vi "emi_SMLoop Start.vi"(5 "Loop ID":i32, 9 "error in (no error)":errorcluster, 12 "Force Stop(F)":bool) -> (6 "Loop command":T1, 10 "error out":errorcluster, 14 "Loop ID out":i32)   [LabVIEW 2011]
uses:
  Private/_emi_ SMLoop sates.ctl
  Loop control/Private/_emi_Loop control int action.ctl
  Private/_emi_ SMLoop restart type.ctl
  S&E reporting/emi_Send S&E Error message.vi
  Basic/0 - General/Error/emi_ Is Error state.vi
  emi_Read System ID.vi
  Private/_emi_GFV System ID.vi
  S&E reporting/Private/_emi_S&E Q Generator.vi
  Loop control/Private/_emi_GFV stop a loop so it can reset.vi
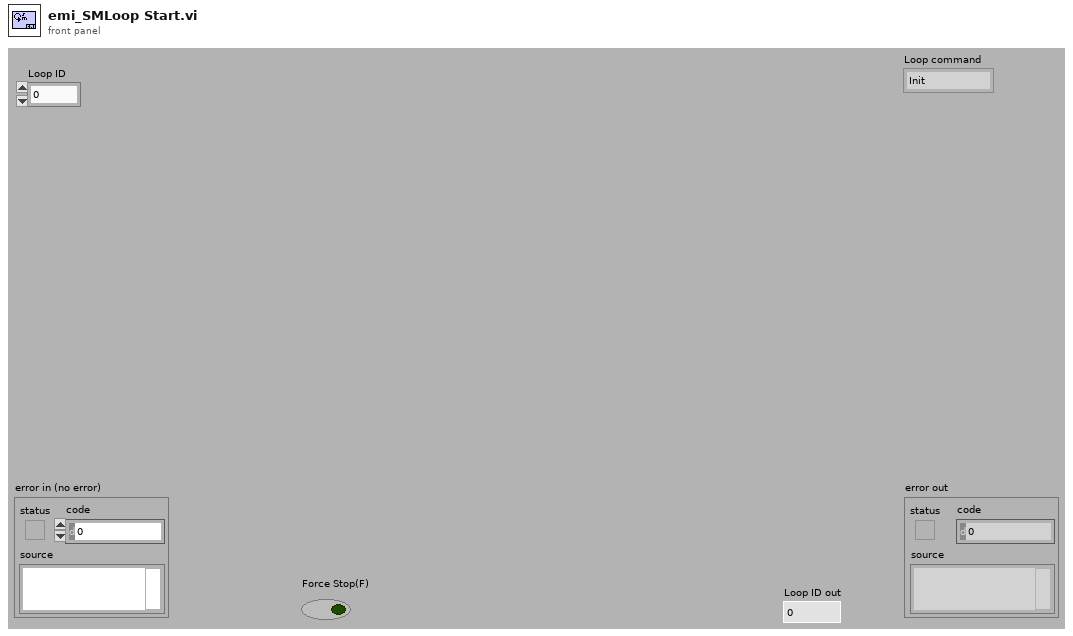
[diagram p1: front panel]
types:
  T1 = typedef "_emi_ SMLoop sates.ctl" = enum16{"Init", "Standby", "Start", "Normal Operation", "Stop", "Error Handling", "End", "Post"}
  T2 = typedef "_emi_ SMLoop restart type.ctl" = enum16{"Normal", "Stop", "Stopped"}
  T3 = typedef "_emi_Loop control int action.ctl" = enum16{"Init index", "Get index", "Set index", "Get Size"}
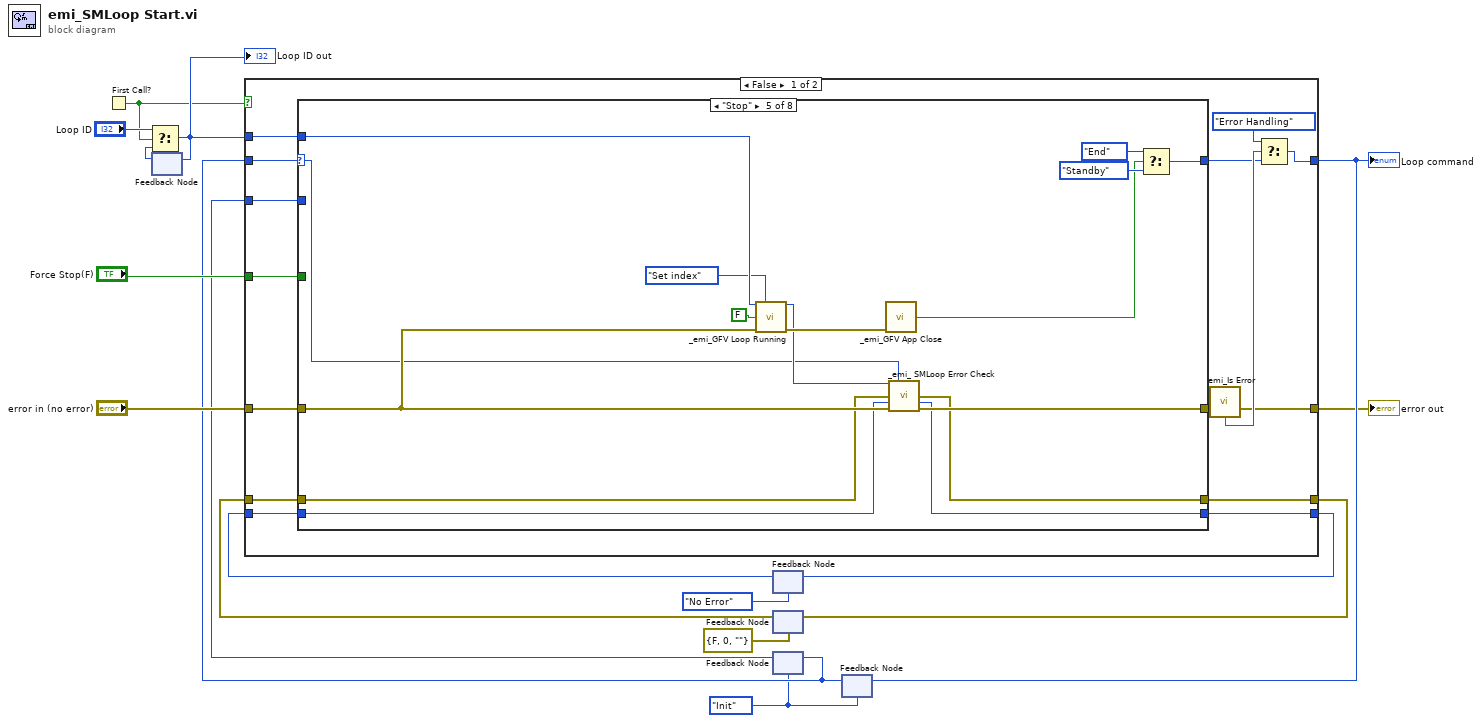
[diagram p0: block diagram]
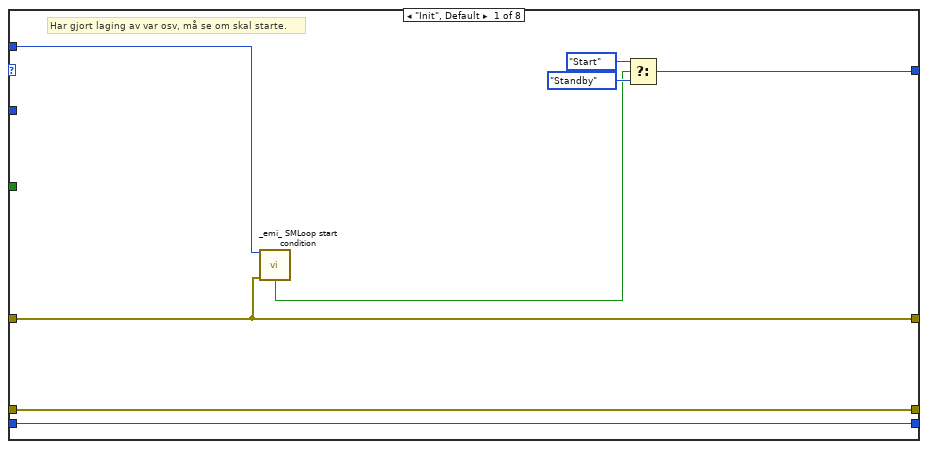
[diagram p2: hidden frame]
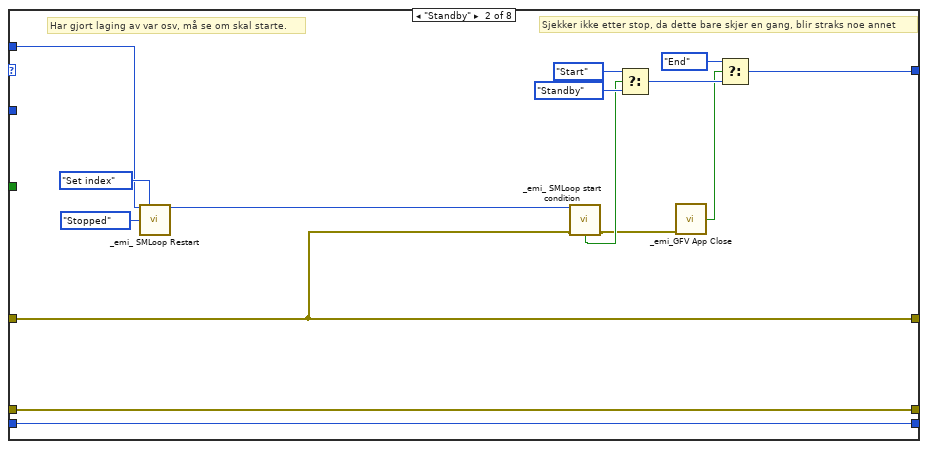
[diagram p3: hidden frame]
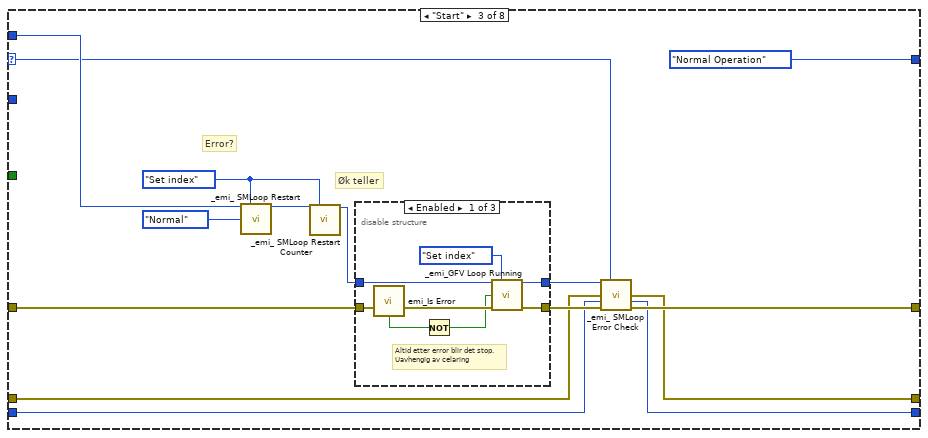
[diagram p4: hidden frame]
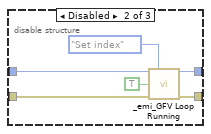
[diagram p5: hidden frame]
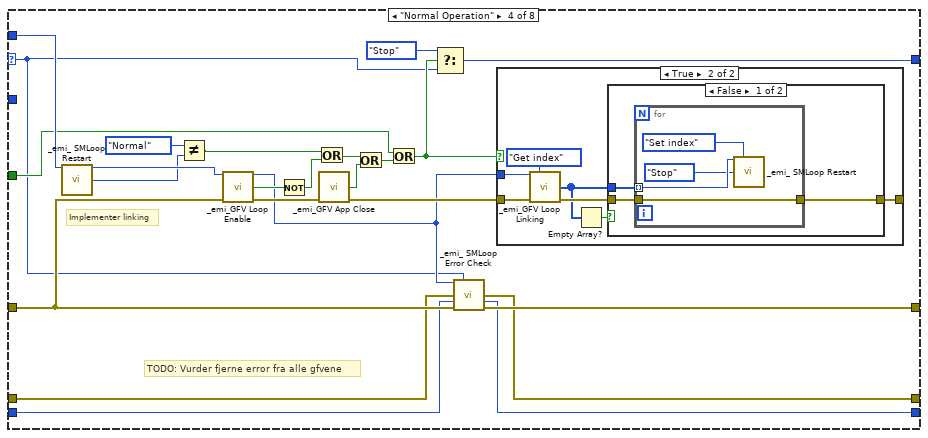
[diagram p7: hidden frame]
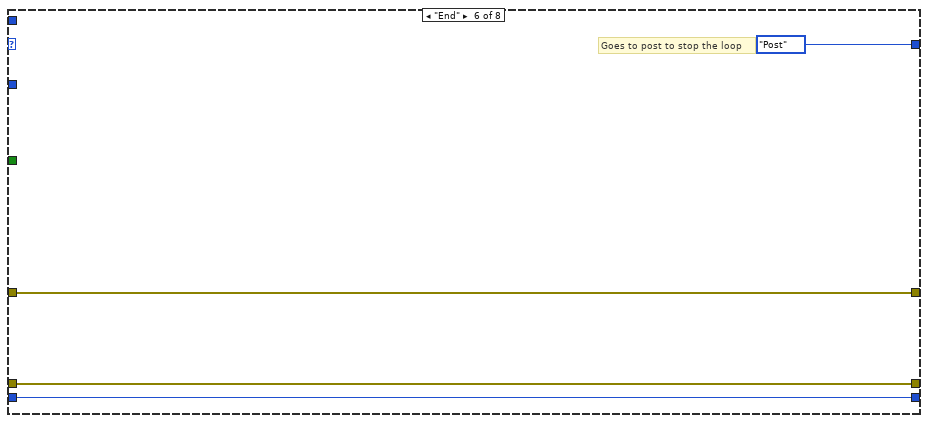
[diagram p10: hidden frame]
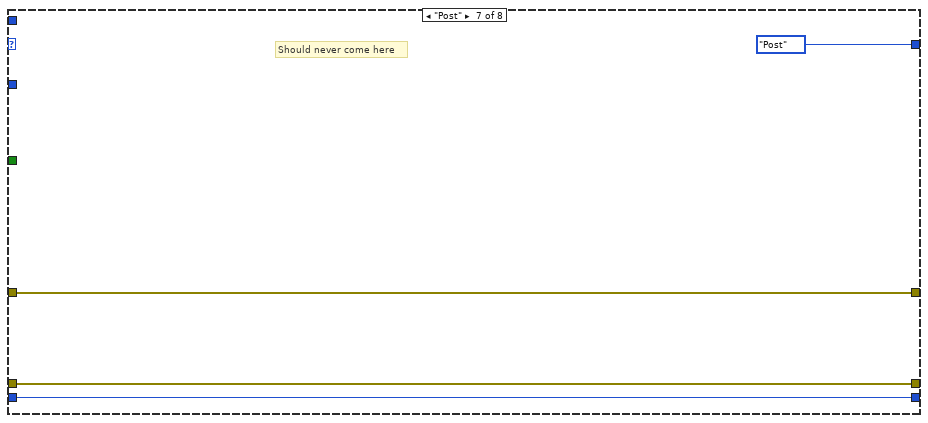
[diagram p11: hidden frame]
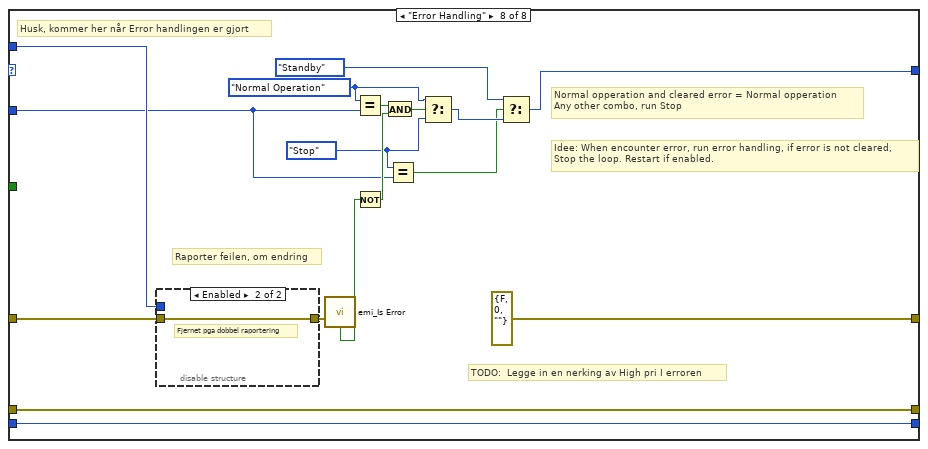
[diagram p12: hidden frame]
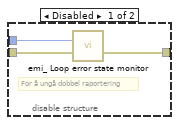
[diagram p13: hidden frame]
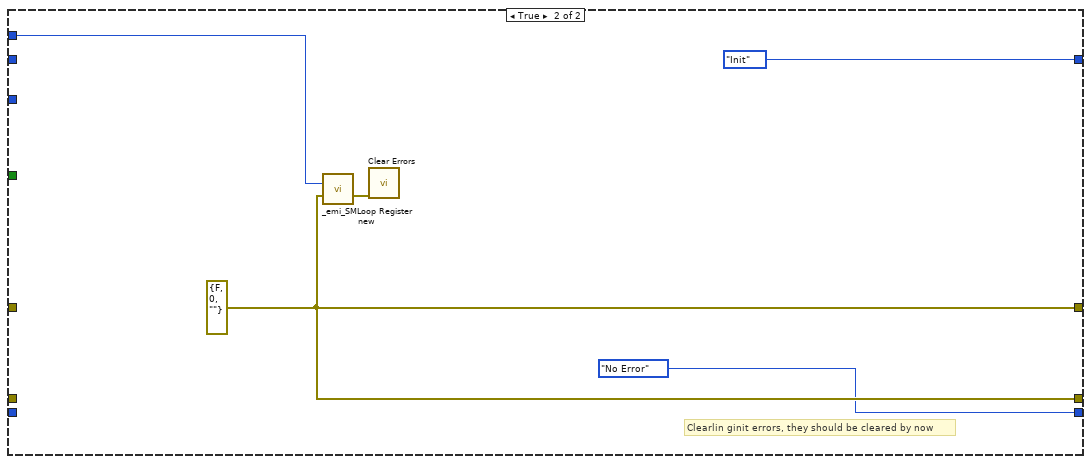
[diagram p14: hidden frame]
diagram:
  w7 = _emi__SMLoop_sates."Init" ("Loop command")
  n1 = First Call?() -> (First Call?: T/F=w13:bool)
  n2 = feedback #1() -> (w17:i32)  [unwired: 1 in]
  n3 = Select(t="Loop ID", s=w13, f=w17) -> (s? t:f=w14:i32)
  "Loop ID out" <- w14
  n4 = feedback-in #1(w14) -> ()
  n5 = feedback #2(enum16{"No Error", "Start", "Normal", "Stop"}."No Error" ("Source Out")) -> (w3:enum16{"No Error", "Start", "Normal", "Stop"})
  n6 = feedback #3(errorcluster {"status"=FALSE, "code"=0, "source"=""} ("Loop Error state out")) -> (w4:errorcluster)
  n7 = feedback #4(w7) -> (w8:T1)
  n8 = feedback #5(w7) -> (w9:T1)
  n9 = case shown="False" w13 {
    tunnel: [w26 _emi__SMLoop_sates."Init" ("Loop command")] -> w16
    tunnel: w9 -> [w22 _]
    tunnel: w14 -> [w31 w175]
    tunnel: [w23 w173] -> w12
    tunnel: "error in (no error)" -> [w32 _]
    tunnel: "Force Stop(F)" -> [w30 _]
    tunnel: w8 -> [w29 _]
    tunnel: [w21 w173] -> w6
    tunnel: [w20 enum16{"No Error", "Start", "Normal", "Stop"}."No Error" ("Source Out")] -> w5
    tunnel: w4 -> [w19 _]
    tunnel: w3 -> [w18 _]
    frame False {
      n10 = case shown="\"Stop\"" w22 {
        selector: w22 -> [_ _ w64 w87 w127 _ _ _]
        tunnel: [w35 w46 w65 w93 w133 w146 w150 errorcluster {"status"=FALSE, "code"=0, "source"=""} ("error out")] -> w24
        tunnel: w32 -> [w35 w46 w68 w94 w134 w146 w150 w167]
        tunnel: [w39 w53 _emi__SMLoop_sates."Normal Operation" ("t") w102 w142 _emi__SMLoop_sates."Post" ("t") _emi__SMLoop_sates."Post" ("t") w155] -> w25
        tunnel: w31 -> [w37 w47 w67 w101 w137 _ _ w164]
        tunnel: w30 -> [_ _ _ w95 _ _ _ _]
        tunnel: w29 -> [_ _ _ _ _ _ _ w154]
        tunnel: [w34 w42 w62 w89 w129 w144 w148 w152] -> w21
        tunnel: [w33 w41 w61 w91 w130 w143 w147 w151] -> w20
        tunnel: w19 -> [w34 w42 w59 w90 w131 w144 w148 w152]
        tunnel: w18 -> [w33 w41 w60 w92 w132 w143 w147 w151]
        frame "Init", Default {
          # "Har gjort laging av var osv, må se om skal starte."
          n11 = call "_emi_ SMLoop start condition.vi"("Loop ID in"=w37, "error in (no error)"=w35) -> ("Klar til start"=w36:bool)  [unwired: 11 in, 2 out]
          n12 = Select(t=_emi__SMLoop_sates."Start", s=w36, f=_emi__SMLoop_sates."Standby") -> (s? t:f=w39:T1)
        }
        frame "Standby" {
          # "Sjekker ikke etter stop, da dette bare skjer en gang, blir straks noe annet"
          # "Har gjort laging av var osv, må se om skal starte."
          n13 = call "_emi_ SMLoop Restart.vi"("Loop Index/Numb"=w47, "Action(Get Index)"=_emi_Loop_control_int_action."Set index", "Value"=_emi__SMLoop_restart_type."Stopped") -> ("Index out"=w45:u16)  [unwired: 10 in, 2 out]
          n14 = call "_emi_ SMLoop start condition.vi"("Loop ID in"=w45, "error in (no error)"=w46) -> ("Klar til start"=w44:bool, "error out"=w43:errorcluster)  [unwired: 11 in, 1 out]
          n15 = Select(t=_emi__SMLoop_sates."Start", s=w44, f=_emi__SMLoop_sates."Standby") -> (s? t:f=w52:T1)
          n16 = call "_emi_GFV App Close.vi"("error in (no error)"=w43) -> ("App Close out"=w50:bool)  [unwired: 13 in, 1 out]
          n17 = Select(t=_emi__SMLoop_sates."End", s=w50, f=w52) -> (s? t:f=w53:T1)
        }
        frame "Start" {
          w56 = _emi_Loop_control_int_action."Set index" ("Action(Get Index)")
          # "Øk teller"
          # "Error?"
          n18 = call "_emi_ SMLoop Restart.vi"("Loop Index/Numb"=w67, "Action(Get Index)"=w56, "Value"=_emi__SMLoop_restart_type."Normal") -> ("Index out"=w58:u16)  [unwired: 10 in, 2 out]
          n19 = call "_emi_ SMLoop Restart Counter.vi"("Loop Index/Numb"=w58, "Action(Get Index)"=w56) -> ("Index out"=w57:u16)  [unwired: 11 in, 2 out]
          n20 = disable-structure shown="Enabled" {
            disable-tunnel: w68 -> [w74 w84 w86]
            disable-tunnel: [w78 w81 w86] -> w66
            disable-tunnel: [w77 w80 w85] -> w63
            disable-tunnel: w57 -> [w76 w79 w85]
            frame Enabled {
              # "Altid etter error blir det stop.\nUavhengig av celaring"
              n21 = call "emi_Is Error.vi"("error in (no error)"=w74) -> ("error out"=w72:errorcluster, "Is Error"=w73:bool)  [unwired: 13 in]
              n22 = Not(x=w73) -> (.not. x?=w71:bool)
              n23 = call "_emi_GFV Loop Running.vi"("Loop Index/Numb"=w76, "Action(Get Index)"=_emi_Loop_control_int_action."Set index", "Loop Running In(F)"=w71, "error in (no error)"=w72) -> ("Index out"=w77:u16, "error out"=w78:errorcluster)  [unwired: 8 in, 2 out]
            }
            frame Disabled {
              n24 = call "_emi_GFV Loop Running.vi"("Loop Index/Numb"=w79, "Action(Get Index)"=_emi_Loop_control_int_action."Set index", "Loop Running In(F)"=TRUE, "error in (no error)"=w84) -> ("Index out"=w80:u16, "error out"=w81:errorcluster)  [unwired: 8 in, 2 out]
            }
            frame Disabled {
              # "Viste Connected når restartet på feil"
            }
          }
          n25 = call "_emi_ SMLoop Error Check.vi"("Loop Index"=w63, "Command ID"=w64, "Loop  Current Error State"=w59, "Current Loop Error/Warning Source"=w60, "Error in"=w66) -> ("Loop Error state out"=w62:errorcluster, "Source Out"=w61:enum16{"No Error", "Start", "Normal", "Stop"}, "error out"=w65:errorcluster)  [unwired: 7 in, 1 out]
        }
        frame "Normal Operation" {
          # "TODO: Vurder fjerne error fra alle gfvene"
          # "Implementer linking"
          n26 = call "_emi_ SMLoop Restart.vi"("Loop Index/Numb"=w101) -> ("Index out"=w100:u16, "Value out"=w98:T2)  [unwired: 12 in, 1 out]
          n27 = Not Equal?(x=_emi__SMLoop_restart_type."Normal", y=w98) -> (x != y?=w99:bool)
          n28 = call "_emi_GFV Loop Enable.vi"("Loop Index/Numb"=w100, "error in (no error)"=w94) -> ("Index out"=w88:u16, "Loop Enable Out"=w107:bool, "error out"=w109:errorcluster)  [unwired: 10 in, 1 out]
          n29 = Not(x=w107) -> (.not. x?=w105:bool)
          n30 = Or(x=w99, y=w105) -> (x .or. y?=w106:bool)
          n31 = call "_emi_GFV App Close.vi"("error in (no error)"=w109) -> ("App Close out"=w110:bool, "error out"=w96:errorcluster)  [unwired: 13 in]
          n32 = Or(x=w106, y=w110) -> (x .or. y?=w108:bool)
          n33 = Or(x=w95, y=w108) -> (x .or. y?=w103:bool)
          n34 = Select(t=_emi__SMLoop_sates."Stop", s=w103, f=w87) -> (s? t:f=w102:T1)
          n35 = call "_emi_ SMLoop Error Check.vi"("Loop Index"=w88, "Command ID"=w87, "Loop  Current Error State"=w90, "Current Loop Error/Warning Source"=w92, "Error in"=w94) -> ("Loop Error state out"=w89:errorcluster, "Source Out"=w91:enum16{"No Error", "Start", "Normal", "Stop"}, "error out"=w93:errorcluster)  [unwired: 7 in, 1 out]
          n36 = case shown="True" w103 {
            tunnel: [w111 w114] -> _
            tunnel: w96 -> [w111 w113]
            tunnel: w88 -> [_ w112]
            frame False {
            }
            frame True {
              n37 = call "_emi_GFV Loop Linking.vi"("Loop Index/Numb"=w112, "Action(Get Index)"=_emi_Loop_control_int_action."Get index", "error in (no error)"=w113) -> ("Linked indexes out"=w115:u16[], "error out"=w116:errorcluster)  [unwired: 9 in, 2 out]
              n38 = Empty Array?(array=w115) -> (empty?=w117:bool)
              n39 = case shown="False" w117 {
                tunnel: w116 -> [w121 w126]
                tunnel: [w120 w126] -> w114
                tunnel: w115 -> [w119 _]
                frame False {
                  n40 = for {
                    tunnel: w121 -> [w124]
                    tunnel: [w124] -> w120
                    tunnel: w119 -> [w123] mode=indexing
                    n41 = call "_emi_ SMLoop Restart.vi"("Loop Index/Numb"=w123, "Action(Get Index)"=_emi_Loop_control_int_action."Set index", "Value"=_emi__SMLoop_restart_type."Stop") -> ()  [unwired: 10 in, 3 out]
                  }
                }
                frame True {
                  # "Empty"
                }
              }
            }
          }
        }
        frame "Stop" {
          n42 = call "_emi_GFV Loop Running.vi"("Loop Index/Numb"=w137, "Action(Get Index)"=_emi_Loop_control_int_action."Set index", "Loop Running In(F)"=FALSE, "error in (no error)"=w134) -> ("Index out"=w128:u16, "error out"=w135:errorcluster)  [unwired: 8 in, 2 out]
          n43 = call "_emi_GFV App Close.vi"("error in (no error)"=w135) -> ("App Close out"=w139:bool)  [unwired: 13 in, 1 out]
          n44 = call "_emi_ SMLoop Error Check.vi"("Loop Index"=w128, "Command ID"=w127, "Loop  Current Error State"=w131, "Current Loop Error/Warning Source"=w132, "Error in"=w134) -> ("Loop Error state out"=w129:errorcluster, "Source Out"=w130:enum16{"No Error", "Start", "Normal", "Stop"}, "error out"=w133:errorcluster)  [unwired: 7 in, 1 out]
          n45 = Select(t=_emi__SMLoop_sates."End", s=w139, f=_emi__SMLoop_sates."Standby") -> (s? t:f=w142:T1)
        }
        frame "End" {
          # "Goes to post to stop the loop"
        }
        frame "Post" {
          # "Should never come here"
        }
        frame "Error Handling" {
          w159 = _emi__SMLoop_sates."Stop" ("f")
          w158 = _emi__SMLoop_sates."Normal Operation" ("x")
          # "Husk, kommer her når Error handlingen er gjort"
          # "Raporter feilen, om endring"
          # "TODO:  Legge in en nerking av High pri I erroren"
          # "Idee: When encounter error, run error handling, if error is not cleared,\nStop the loop. Restart if enabled."
          # "Normal opperation and cleared error = Normal opperation\nAny other combo, run Stop"
          n46 = disable-structure shown="Enabled" {
            disable-tunnel: w167 -> [w170 w171]
            disable-tunnel: [w169 w171] -> w165
            disable-tunnel: w164 -> [w168 _]
            frame Disabled {
              # "For å ungå dobbel raportering"
              n47 = call "emi_ Loop error state monitor.vi"("Loop ID in"=w168, "error in (no error)"=w170) -> ("error out"=w169:errorcluster)  [unwired: 12 in, 1 out]
            }
            frame Enabled {
              # "Fjernet pga dobbel raportering"
            }
          }
          n48 = call "emi_Is Error.vi"("error in (no error)"=w165) -> ("Is Error"=w153:bool)  [unwired: 13 in, 1 out]
          n49 = Equal?(x=w158, y=w154) -> (x = y?=w157:bool)
          n50 = Not(x=w153) -> (.not. x?=w160:bool)
          n51 = And(x=w157, y=w160) -> (x .and. y?=w156:bool)
          n52 = Equal?(x=w159, y=w154) -> (x = y?=w161:bool)
          n53 = Select(t=w158, s=w156, f=w159) -> (s? t:f=w162:T1)
          n54 = Select(t=_emi__SMLoop_sates."Standby", s=w161, f=w162) -> (s? t:f=w155:T1)
        }
      }
      n55 = call "emi_Is Error.vi"("error in (no error)"=w24) -> ("error out"=w23:errorcluster, "Is Error"=w27:bool)  [unwired: 13 in]
      n56 = Select(t=_emi__SMLoop_sates."Error Handling", s=w27, f=w25) -> (s? t:f=w26:T1)
    }
    frame True {
      w173 = errorcluster {"status"=FALSE, "code"=0, "source"=""} ("error in (no error)")
      # "Clearlin ginit errors, they should be cleared by now"
      n57 = call "_emi_SMLoop Register new.vi"("Loop ID"=w175, "error in (no error)"=w173) -> ("error out"=w174:errorcluster)  [unwired: 12 in, 1 out]
      n58 = call <vilib>:"Clear Errors.vi"("error in (no error)"=w174) -> ()  [unwired: 6 in, 1 out]
    }
  }
  "error out" <- w12
  "Loop command" <- w16
  n59 = feedback-in #2(w5) -> ()
  n60 = feedback-in #3(w6) -> ()
  n61 = feedback-in #4(w9) -> ()
  n62 = feedback-in #5(w16) -> ()
